vi "Add Plot.vi"(0 "Display State In":T2, 1 "visible":bool, 2 "cursor":bool, 3 "Y0":dbl, 5 "plot":cluster{"X":dbl[], "Y":dbl[]}, 7 "name":string, 9 "Container State":T6, 10 "labpos":T1={"Index"=-1, "Xoff"=nan, "Yoff"=nan}, 11 "error in (no error)":errorcluster, 12 "color":u32(colorbox)=16777216, 13 "style":enum16{"Normal", "Highlight", "Shadow"}(ring)) -> (4 "Display State Out":T2, 14 "color out":u32(colorbox), 15 "error out":errorcluster)   [LabVIEW 2015, in "Interactive Graph.xctl"]
uses:
  Interactive Graph.xctl
  <vilib>/_xctls/Container State.ctl
  State.vi
  Persistent.ctl
  Plot.ctl
  EPhys/LV Source/Work Panel VIs/Typedefs/EPhysWork-Label Position.ctl
  Events.ctl
  Selection.ctl
  XRange.ctl
  YScale.ctl
  Cursor.ctl
  <vilib>/Analysis/baseanly.llb/Mean (DBL).vi
  <vilib>/Analysis/NI_AALBase.lvlib
  <vilib>/_xctls/XControlSupport.lvlib
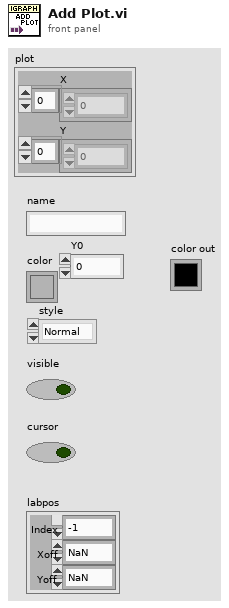
[diagram p1: front panel]
types:
  T1 = typedef "EPhysWork-Label Position.ctl" = cluster{"Index":i32, "Xoff":dbl, "Yoff":dbl}
  T2 = typedef "Interactive Graph.xctl/State.vi" = cluster{"ref":refnum<vi>, "actions":string[], "Persist":T3, "cursor":bool, "prescale":dbl, "palette":u32[], "colIndex":i32, "to add":T4, "Events":T5, "selected":i32, "to show":cluster{"Visible":bool, "Start":i32, "Length":i32}, "maxplot":i32, "Y0":dbl[], "plotnum":i32}
  T3 = typedef "Interactive Graph.xctl/Persistent.ctl" = cluster{"Scale":dbl, "Xrange":cluster{"min":dbl, "max":dbl}}
  T4 = typedef "Interactive Graph.xctl/Plot.ctl" = cluster{"plot":cluster{"X":dbl[], "Y":dbl[]}, "name":string, "Y0":dbl, "color":u32, "Style":enum16{"Normal", "Highlight", "Shadow"}, "labpos":T1, "visible":bool, "cursor":bool}
  T5 = typedef "Interactive Graph.xctl/Events.ctl" = cluster{"Selection":refnum<user-event>, "XRange":refnum<user-event>, "YScale":refnum<user-event>, "CursorPos":refnum<user-event>}
  T6 = typedef "XControlSupport.lvlib/Container State.ctl" = cluster{"Indicator?":bool, "Run Mode?":bool, " Refnum":refnum<vi>}
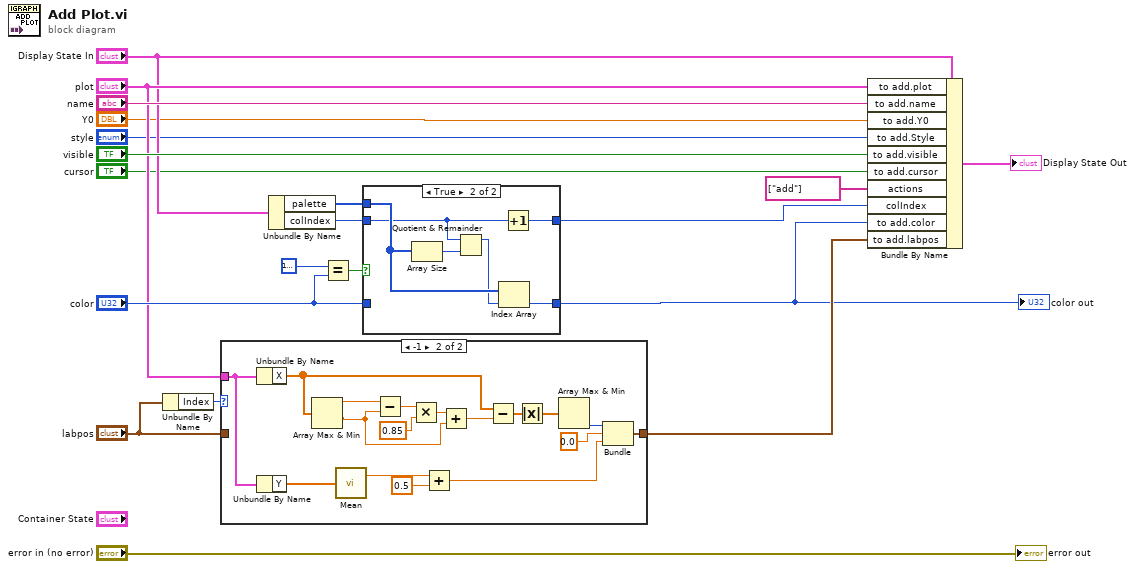
[diagram p0: block diagram]
diagram:
  n1 = Unbundle By Name("labpos") -> ("Index"=w7:i32)
  n2 = case shown="-1" w7 {
    tunnel: "plot" -> [_ w35]
    tunnel: "labpos" -> [w21 _]
    tunnel: [w21 w22] -> w5
    frame 0, Default {
    }
    frame -1 {
      n3 = Unbundle By Name(w35) -> ("X"=w28:dbl[])
      n4 = Unbundle By Name(w35) -> ("Y"=w38:dbl[])
      n5 = Array Max & Min(array=w28) -> (max value=w27:dbl, min value=w26:dbl)  [unwired: 2 out]
      n6 = call-poly <vilib>:"Mean.vi"("X"=w38) -> ("mean"=w37:dbl)  [unwired: 1 out]
      n7 = Subtract(x=w27, y=w26) -> (x-y=w34:dbl)
      n8 = Multiply(x=w34, y=0.85) -> (x*y=w32:dbl)
      n9 = Add(x=w37, y=0.5) -> (x+y=w23:dbl)
      n10 = Add(x=w32, y=w26) -> (x+y=w31:dbl)
      n11 = Subtract(x=w28, y=w31) -> (x-y=w30:dbl[])
      n12 = Absolute Value(x=w30) -> (abs(x)=w29:dbl[])
      n13 = Array Max & Min(array=w29) -> (min index (indices)=w24:i32)  [unwired: 3 out]
      n14 = Bundle(w24, "to add.labpos.Xoff"=0.0, w23) -> (w22:cluster{i32, "to add.labpos.Xoff":dbl, dbl})  [unwired: 1 in]
    }
  }
  n15 = Unbundle By Name("Display State In") -> ("palette"=w12:u32[], "colIndex"=w13:i32)
  n16 = Equal?(x=u32 16777216, y="color") -> (x = y?=w15:bool)
  n17 = case shown="True" w15 {
    tunnel: "color" -> [w40 _]
    tunnel: [w40 w44] -> w1
    tunnel: [w39 w41] -> w2
    tunnel: w13 -> [w39 w42]
    tunnel: w12 -> [_ w45]
    frame False {
    }
    frame True {
      n18 = Array Size(array=w45) -> (size(s)=w46:i32)
      n19 = Quotient & Remainder(x=w42, y=w46) -> (x-y*floor(x/y)=w43:i32)  [unwired: 1 out]
      n20 = Index Array(array=w45, index=w43) -> (element=w44:u32)
      n21 = Increment(x=w42) -> (x+1=w41:i32)
    }
  }
  "color out" <- w1
  n22 = Bundle By Name(cluster="Display State In", "to add.plot"="plot", "to add.name"="name", "to add.Y0"="Y0", "to add.Style"="style", "to add.visible"="visible", "to add.cursor"="cursor", "actions"=string[] ["add"], "colIndex"=w2, "to add.color"=w1, "to add.labpos"=w5) -> (→"Display State Out":T2)
  "error out" <- "error in (no error)"
